vi "SendProcessEnded.vi"(8 "error in (no error)":errorcluster, 11 "Process Refnum":refnum<vi>) -> (0 "error out":errorcluster)   [LabVIEW 2011]
uses:
  030 - EVENTS/EnumFgvEventCommand.ctl
  030 - EVENTS/05 - FromProcesses/FromProcessEvent.ctl
  030 - EVENTS/05 - FromProcesses/FromProcessesEventType.ctl
  030 - EVENTS/03 - ToMessageHandlerProcess/ToMessageHandlerEvent.ctl
  030 - EVENTS/03 - ToMessageHandlerProcess/enumMessageCriticity.ctl
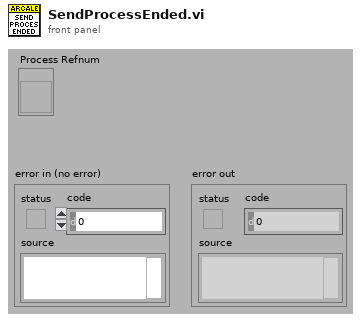
[diagram p1: front panel]
types:
  T1 = typedef "FromProcessesEventType.ctl" = enum16{"Started", "Autotest", "Ended"}
  T2 = typedef "FromProcessEvent.ctl" = cluster{"Command":T1, "Process path":path, "Message":T3, "Process Refnum":refnum<vi>}
  T3 = typedef "ToMessageHandlerEvent.ctl" = cluster{"date / time":timestamp, "Criticity":T4, "Emitter":string, "Message":string}
  T4 = typedef "enumMessageCriticity.ctl" = enum16{"No error", "Info", "Warning", "Error", "Fatal error"}
  T5 = typedef "EnumFgvEventCommand.ctl" = enum16{"Setup", "Cleanup", "Get"}
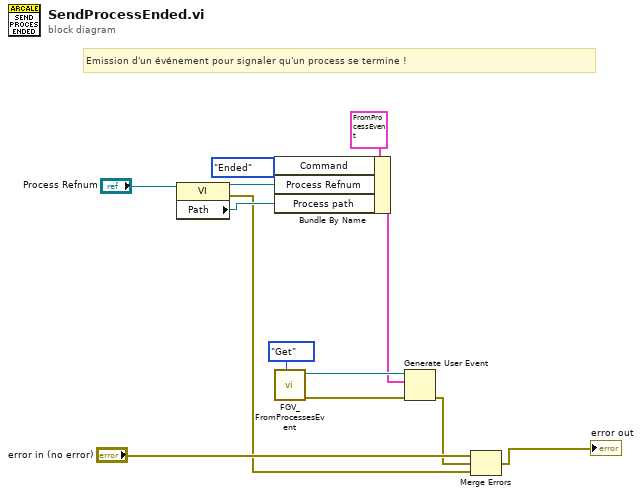
[diagram p0: block diagram]
diagram:
  # "Emission d'un événement pour signaler qu'un process se termine !"
  n1 = property class="VI"(reference="Process Refnum") -> (reference out=w2:refnum<vi>, error out=w1:errorcluster, "Path"=w3:path)  [unwired: 1 in]
  n2 = Bundle By Name(cluster=T2 {"Command"=enum."Started", "Process path"=path "", "Message"={"date / time"=timestamp(0 s since 1904-01-01), "Criticity"=enum."No error", "Emitter"="", "Message"=""}, "Process Refnum"=refnum} ("event data"), "Command"=FromProcessesEventType."Ended", "Process Refnum"=w2, "Process path"=w3) -> (w9:T2)
  n3 = call "FGV_FromProcessesEvent.vi"("Command"=EnumFgvEventCommand."Get") -> ("error out"=w12:errorcluster, "From Process Event"=w11:refnum<user-event>)  [unwired: 9 in]
  n4 = Generate User Event(user event=w11, event data cluster=w9, error in=w12) -> (error out=w6:errorcluster)  [unwired: 1 out]
  n5 = Merge Errors("error in (no error)", w6, w1) -> (→"error out":errorcluster)
